vi "ScanListParse.vi"(11 "Input":string="SCANALL") -> (3 "Output":string[](array[string]))   [LabVIEW 2019]
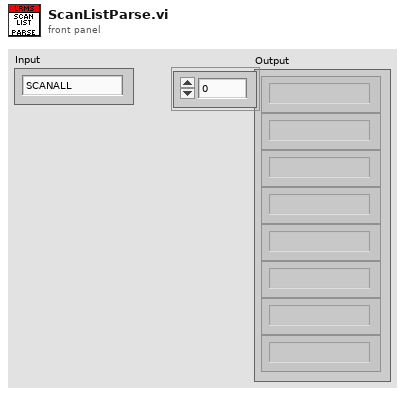
[diagram p1: front panel]
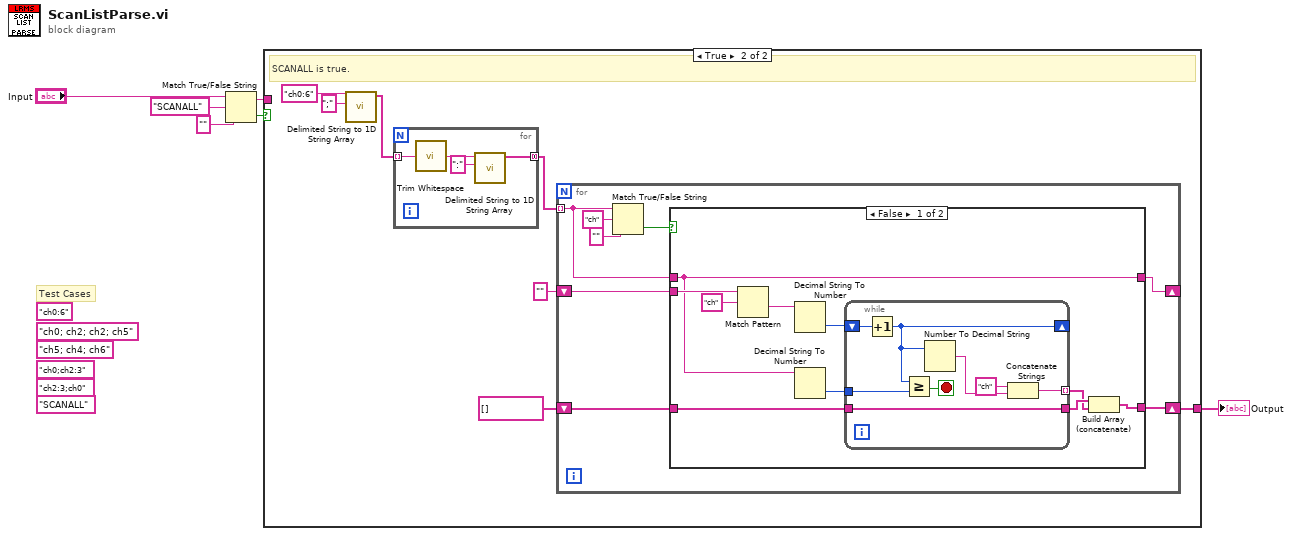
[diagram p0: block diagram]
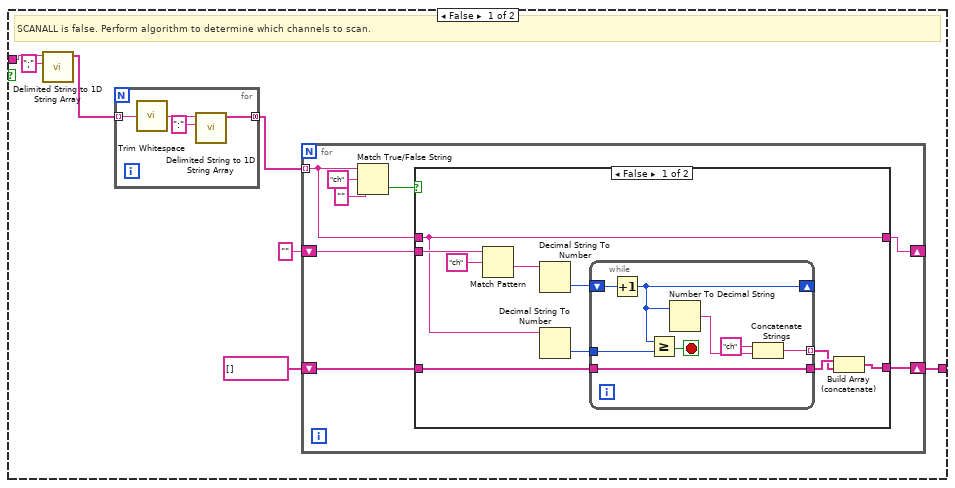
[diagram p2: hidden frame]
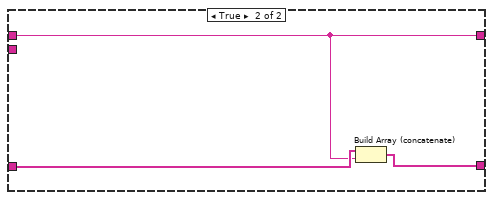
[diagram p3: hidden frame]
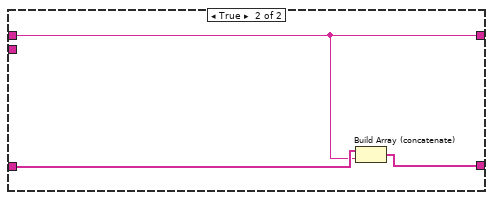
[diagram p4: hidden frame]
diagram:
  (unwired) "SCANALL" ("Input 2")
  (unwired) "ch5; ch4; ch6"
  (unwired) "ch0; ch2; ch2; ch5"
  (unwired) "ch0:6"
  (unwired) "ch2:3;ch0"
  (unwired) "ch0;ch2:3"
  # "Test Cases"
  n1 = Match True/False String(2:"" ("false string"), 3:"SCANALL" ("true string"), 4:"Input") -> (0:w2:bool, 1:w3:string)
  n2 = case shown="True" w2 {
    tunnel: [w8 w48] -> w6
    tunnel: w3 -> [w7 _]
    frame False {
      # "SCANALL is false. Perform algorithm to determine which channels to scan."
      n3 = call <vilib>:"Delimited String to 1D String Array.vi"("delimiter"=";", "delimited string"=w7) -> ("string array"=w12:string[])  [unwired: 9 in]
      n4 = for {
        tunnel: w12 -> [w45] mode=indexing
        tunnel: [w44] -> w11 mode=concatenating
        n5 = call <vilib>:"Trim Whitespace.vi"("string"=w45) -> ("trimmed string"=w43:string)  [unwired: 1 in]
        n6 = call <vilib>:"Delimited String to 1D String Array.vi"("delimiter"=":", "delimited string"=w43) -> ("string array"=w44:string[])  [unwired: 9 in]
      }
      n7 = for {
        tunnel: w11 -> [w18] mode=indexing
        shift-right: [w15] -> _
        shift-left: "" ("String") -> [w17]
        shift-right: [w14] -> w8
        shift-left: string[] [] -> [w16]
        n8 = Match True/False String(2:"" ("false string"), 3:"ch" ("true string"), 4:w18) -> (0:w19:bool)  [unwired: 1 out]
        n9 = case shown="False" w19 {
          tunnel: w18 -> [w28 w40]
          tunnel: [w28 w40] -> w15
          tunnel: w17 -> [w30 _]
          tunnel: [w24 w42] -> w14
          tunnel: w16 -> [w25 w41]
          frame False {
            n10 = Match Pattern(string=w30, regular expression="ch") -> (after substring=w29:string)  [unwired: 1 in, 3 out]
            n11 = Decimal String To Number(string=w29) -> (number=w26:i32)  [unwired: 2 in, 1 out]
            n12 = Decimal String To Number(string=w28) -> (number=w27:i32)  [unwired: 2 in, 1 out]
            n13 = while {
              tunnel: [w36] -> w22 mode=indexing
              tunnel: w25 -> [w32]
              shift-right: [w33] -> _
              shift-left: w26 -> [w34]
              tunnel: w27 -> [w35]
              tunnel: [w32] -> w23
              stop <- w39 stop-if-true
              n14 = Increment(x=w34) -> (x+1=w33:i32)
              n15 = Greater Or Equal?(x=w33, y=w35) -> (x >= y?=w39:bool)
              n16 = Number To Decimal String(number=w33) -> (decimal integer string=w37:string)  [unwired: 1 in]
              n17 = Concatenate Strings("ch" ("element"), w37) -> (w36:string)
            }
            n18 = Build Array (concatenate)(w23, w22) -> (w24:string[])
          }
          frame True {
            n19 = Build Array (concatenate)(w41, w40) -> (w42:string[])
          }
        }
      }
    }
    frame True {
      # "SCANALL is true."
      n20 = call <vilib>:"Delimited String to 1D String Array.vi"("delimiter"=";", "delimited string"="ch0:6") -> ("string array"=w52:string[])  [unwired: 9 in]
      n21 = for {
        tunnel: w52 -> [w85] mode=indexing
        tunnel: [w84] -> w51 mode=concatenating
        n22 = call <vilib>:"Trim Whitespace.vi"("string"=w85) -> ("trimmed string"=w83:string)  [unwired: 1 in]
        n23 = call <vilib>:"Delimited String to 1D String Array.vi"("delimiter"=":", "delimited string"=w83) -> ("string array"=w84:string[])  [unwired: 9 in]
      }
      n24 = for {
        tunnel: w51 -> [w58] mode=indexing
        shift-right: [w55] -> _
        shift-left: "" ("String") -> [w57]
        shift-right: [w54] -> w48
        shift-left: string[] [] -> [w56]
        n25 = Match True/False String(2:"" ("false string"), 3:"ch" ("true string"), 4:w58) -> (0:w59:bool)  [unwired: 1 out]
        n26 = case shown="False" w59 {
          tunnel: w58 -> [w68 w80]
          tunnel: [w68 w80] -> w55
          tunnel: w57 -> [w70 _]
          tunnel: [w64 w82] -> w54
          tunnel: w56 -> [w65 w81]
          frame False {
            n27 = Match Pattern(string=w70, regular expression="ch") -> (after substring=w69:string)  [unwired: 1 in, 3 out]
            n28 = Decimal String To Number(string=w69) -> (number=w66:i32)  [unwired: 2 in, 1 out]
            n29 = Decimal String To Number(string=w68) -> (number=w67:i32)  [unwired: 2 in, 1 out]
            n30 = while {
              tunnel: [w76] -> w62 mode=indexing
              tunnel: w65 -> [w72]
              shift-right: [w73] -> _
              shift-left: w66 -> [w74]
              tunnel: w67 -> [w75]
              tunnel: [w72] -> w63
              stop <- w79 stop-if-true
              n31 = Increment(x=w74) -> (x+1=w73:i32)
              n32 = Greater Or Equal?(x=w73, y=w75) -> (x >= y?=w79:bool)
              n33 = Number To Decimal String(number=w73) -> (decimal integer string=w77:string)  [unwired: 1 in]
              n34 = Concatenate Strings("ch" ("element"), w77) -> (w76:string)
            }
            n35 = Build Array (concatenate)(w63, w62) -> (w64:string[])
          }
          frame True {
            n36 = Build Array (concatenate)(w81, w80) -> (w82:string[])
          }
        }
      }
    }
  }
  "Output" <- w6
